vi "Launch_Dequeue_Message_FGV.vi"(8 "error in (no error)":errorcluster) -> (0 "error out":errorcluster, 1 "Message Data":variant, 2 "Message":string)   [LabVIEW 2024, in "LaunchTest.lvlib"]
doc: "ThisVI\n------------------------------\nDequeue Message\n------------------------------\n-Dequeue the message"
uses:
  LaunchTest.lvlib
  PrivateControls/Launch_FGV_Queue_Control.ctl
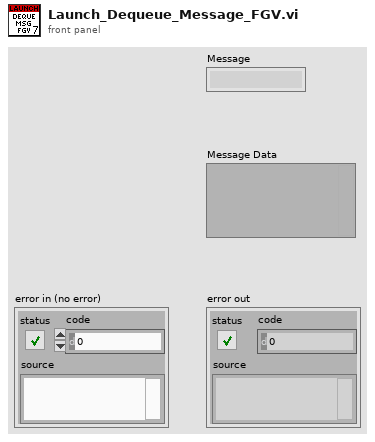
[diagram p1: front panel]
types:
  T1 = typedef "LaunchTest.lvlib/Launch_FGV_Queue_Control.ctl" = enum16{"Release", "Get", "Set", "Flush"}
  T2 = typedef "LaunchTest.lvlib/Launch_Message Queue.lvlib/Launch_Message Cluster.ctl" = cluster{"Message":string, "Message Data":variant}
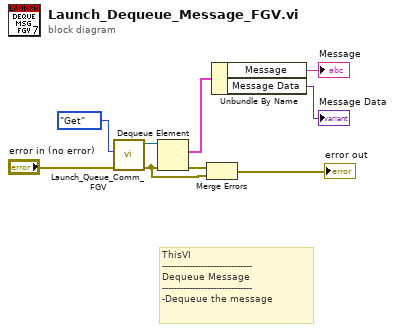
[diagram p0: block diagram]
diagram:
  # "ThisVI\n------------------------------\nDequeue Message\n------------------------------\n-Dequeue the message"
  n1 = call "Launch_Queue_Comm_FGV.vi"("error in (no error)"="error in (no error)", "Enum"=Launch_FGV_Queue_Control."Get") -> ("error Out"=w6:errorcluster, "queue Out"=w3:refnum<queue>)  [unwired: 8 in]
  n2 = Dequeue Element(queue=w3, error in (no error)=w6) -> (element=w4:T2, error out=w5:errorcluster)  [unwired: 1 in, 2 out]
  n3 = Merge Errors(w5, w6) -> (→"error out":errorcluster)
  n4 = Unbundle By Name(w4) -> ("Message"=→"Message":string, "Message Data"=→"Message Data":variant)
